vi "AVS_Read_Ch5-6-7.vi"(11 "refnum":refnum<file>) -> (1 "Resistance reading ch 5":dbl format="%.2f", 2 "Resistance reading ch 7":dbl format="%.2f", 3 "Resistance reading ch 6":dbl format="%.2f")   [LabVIEW 2016]
uses:
  Instrument_Setup_v2.vi
panel:
  in  "Delay (sec) 4":i16=1 min=0 max=3600 step=1
  in  "error in (no error) 5":errorcluster
  in  "error in (no error) 4":errorcluster
  in  "error in (no error) 3":errorcluster
  in  "Delay (sec) 3":i16=1 min=0 max=3600 step=1
  in  "Delay (sec) 2":i16=1 min=0 max=3600 step=1
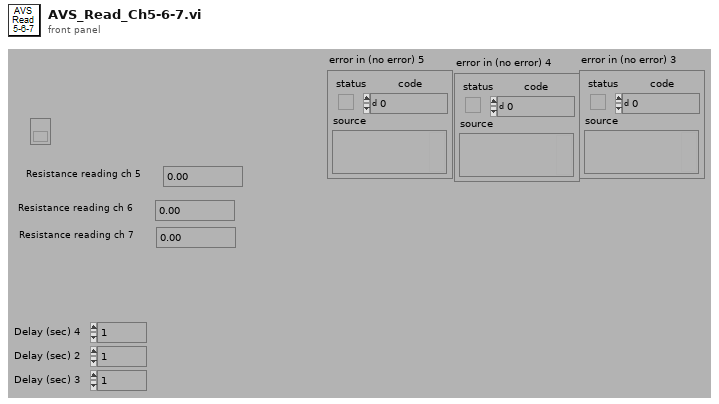
[diagram p1: front panel]
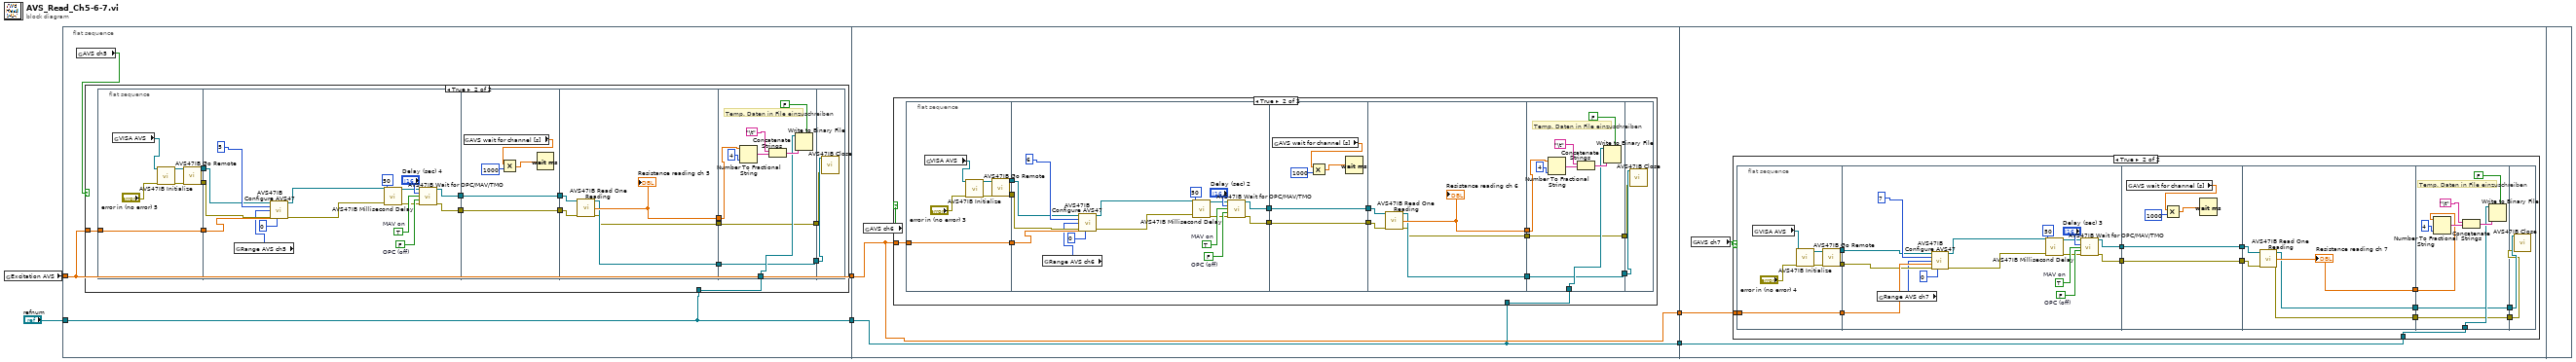
[diagram p0: block diagram]
diagram:
  n1 = global read "Instrument_Setup_v2.vi" "Excitation AVS"() -> (w5:dbl)
  n2 = flat-sequence {
    tunnel: "refnum" -> [w8]
    tunnel: w5 -> [w9]
    tunnel: [w9] -> w2
    tunnel: [w8] -> w1
    tunnel: [w69] -> w6
    tunnel: [w68] -> w3
    tunnel: w2 -> [w69]
    tunnel: w1 -> [w68]
    tunnel: w6 -> [w131]
    tunnel: w3 -> [w129]
    frame #0 {
      n3 = global read "Instrument_Setup_v2.vi" "AVS ch5"() -> (w7:bool)
      n4 = case shown="True" w7 {
        tunnel: w9 -> [_ w19]
        tunnel: w8 -> [_ w17]
        frame False {
        }
        frame True {
          n5 = flat-sequence {
            tunnel: w19 -> [w30]
            tunnel: [w30] -> w16
            tunnel: [w26] -> w15
            tunnel: [w25] -> w14
            tunnel: [w37] -> w23
            tunnel: [w36] -> w22
            tunnel: w16 -> [w34]
            tunnel: w15 -> [w33]
            tunnel: w14 -> [w32]
            tunnel: w23 -> [w51]
            tunnel: w22 -> [w50]
            tunnel: [w51] -> w21
            tunnel: [w50] -> w20
            tunnel: w21 -> [w56]
            tunnel: w20 -> [w55]
            tunnel: [w54] -> w18
            tunnel: [w53] -> w13
            tunnel: [w52] -> w10
            tunnel: w18 -> [w61]
            tunnel: w17 -> [w59]
            tunnel: w13 -> [w58]
            tunnel: [w58] -> w12
            tunnel: [w57] -> w11
            tunnel: w10 -> [w57]
            tunnel: w12 -> [w67]
            tunnel: w11 -> [w66]
            frame #0 {
              n6 = global read "Instrument_Setup_v2.vi" "VISA AVS"() -> (w24:refnum<visa-resource-name>)
              n7 = call "AVS47IB Initialize.vi"("VISA session"=w24, "error in (no error)"="error in (no error) 5") -> ("dup VISA session"=w28:refnum<visa-resource-name>, "error out"=w27:errorcluster)  [unwired: 12 in]
              n8 = call "AVS47IB Go Remote.vi"("VISA session"=w28, "error in (no error)"=w27) -> ("dup VISA session"=w26:refnum<visa-resource-name>, "error out"=w25:errorcluster)  [unwired: 12 in]
            }
            frame #1 {
              w44 = FALSE  # OPC (off)
              w45 = TRUE  # MAV on
              n9 = global read "Instrument_Setup_v2.vi" "Range AVS ch5"() -> (w31:i8)
              n10 = call "AVS47IB Configure AVS47.vi"("VISA session"=w33, "CHANNEL (-1:no change )"=i8 5, "RANGE  (-1:no change)"=w31, "EXCITATION (-1:no change)"=w34, "error in (no error)"=w32, "DISPLAY (-1:no change)"=i8 0) -> ("dup VISA session"=w39:refnum<visa-resource-name>, "error out"=w38:errorcluster)  [unwired: 8 in]
              n11 = call "AVS47IB Millisecond Delay.vi"("VISA session"=w39, "Delay (50 ms)"=50, "error in (no error)"=w38) -> ("dup VISA session"=w42:refnum<visa-resource-name>, "error out"=w41:errorcluster)  [unwired: 11 in]
              n12 = call "AVS47IB Wait for OPC/MAV/TMO.vi"("VISA session"=w42, "Timeout (2 sec)"="Delay (sec) 4", "MAV (on)"=w45, "OPC (off)"=w44, "error in (no error)"=w41) -> ("dup VISA session"=w37:refnum<visa-resource-name>, "error out"=w36:errorcluster)  [unwired: 8 in, 1 out]
            }
            frame #2 {
              n13 = global read "Instrument_Setup_v2.vi" "AVS wait for channel [s]"() -> (w49:dbl)
              n14 = Multiply(x=w49, y=1000) -> (x*y=w47:dbl)
              n15 = Wait (ms)(milliseconds to wait=w47) -> ()  [unwired: 1 out]
            }
            frame #3 {
              n16 = call "AVS47IB Read One Reading.vi"("VISA session"=w56, "error in (no error)"=w55) -> ("dup VISA session"=w53:refnum<visa-resource-name>, "Resistance reading"=w54:dbl, "error out"=w52:errorcluster)  [unwired: 9 in, 2 out]
              "Resistance reading ch 5" <- w54
            }
            frame #4 {
              # "Temp. Daten in File einzuschreiben"
              n17 = Number To Fractional String(number=w61, precision (6)=i16 4) -> (F-format string=w60:string)  [unwired: 2 in]
              n18 = Concatenate Strings("\t", w60) -> (w65:string)
              n19 = Write to Binary File ("Write File")(file (use dialog)=w59, data=w65, 5:FALSE ("prepend array or string size? (T)")) -> ()  [unwired: 3 in, 3 out]
            }
            frame #5 {
              n20 = call "AVS47IB Close.vi"("VISA session"=w67, "error in (no error)"=w66) -> ()  [unwired: 13 in, 1 out]
            }
          }
        }
      }
    }
    frame #1 {
      n21 = global read "Instrument_Setup_v2.vi" "AVS ch6"() -> (w70:bool)
      n22 = case shown="True" w70 {
        tunnel: w69 -> [_ w80]
        tunnel: w68 -> [_ w78]
        frame False {
        }
        frame True {
          n23 = flat-sequence {
            tunnel: w80 -> [w91]
            tunnel: [w91] -> w77
            tunnel: [w87] -> w76
            tunnel: [w86] -> w75
            tunnel: [w98] -> w84
            tunnel: [w97] -> w83
            tunnel: w77 -> [w95]
            tunnel: w76 -> [w94]
            tunnel: w75 -> [w93]
            tunnel: w84 -> [w112]
            tunnel: w83 -> [w111]
            tunnel: [w112] -> w82
            tunnel: [w111] -> w81
            tunnel: w82 -> [w117]
            tunnel: w81 -> [w116]
            tunnel: [w115] -> w79
            tunnel: [w114] -> w74
            tunnel: [w113] -> w71
            tunnel: w79 -> [w122]
            tunnel: w78 -> [w120]
            tunnel: w74 -> [w119]
            tunnel: [w119] -> w73
            tunnel: [w118] -> w72
            tunnel: w71 -> [w118]
            tunnel: w73 -> [w128]
            tunnel: w72 -> [w127]
            frame #0 {
              n24 = global read "Instrument_Setup_v2.vi" "VISA AVS"() -> (w85:refnum<visa-resource-name>)
              n25 = call "AVS47IB Initialize.vi"("VISA session"=w85, "error in (no error)"="error in (no error) 3") -> ("dup VISA session"=w89:refnum<visa-resource-name>, "error out"=w88:errorcluster)  [unwired: 12 in]
              n26 = call "AVS47IB Go Remote.vi"("VISA session"=w89, "error in (no error)"=w88) -> ("dup VISA session"=w87:refnum<visa-resource-name>, "error out"=w86:errorcluster)  [unwired: 12 in]
            }
            frame #1 {
              w105 = FALSE  # OPC (off)
              w106 = TRUE  # MAV on
              n27 = global read "Instrument_Setup_v2.vi" "Range AVS ch6"() -> (w92:i8)
              n28 = call "AVS47IB Configure AVS47.vi"("VISA session"=w94, "CHANNEL (-1:no change )"=i8 6, "RANGE  (-1:no change)"=w92, "EXCITATION (-1:no change)"=w95, "error in (no error)"=w93, "DISPLAY (-1:no change)"=i8 0) -> ("dup VISA session"=w100:refnum<visa-resource-name>, "error out"=w99:errorcluster)  [unwired: 8 in]
              n29 = call "AVS47IB Millisecond Delay.vi"("VISA session"=w100, "Delay (50 ms)"=50, "error in (no error)"=w99) -> ("dup VISA session"=w103:refnum<visa-resource-name>, "error out"=w102:errorcluster)  [unwired: 11 in]
              n30 = call "AVS47IB Wait for OPC/MAV/TMO.vi"("VISA session"=w103, "Timeout (2 sec)"="Delay (sec) 2", "MAV (on)"=w106, "OPC (off)"=w105, "error in (no error)"=w102) -> ("dup VISA session"=w98:refnum<visa-resource-name>, "error out"=w97:errorcluster)  [unwired: 8 in, 1 out]
            }
            frame #2 {
              n31 = global read "Instrument_Setup_v2.vi" "AVS wait for channel [s]"() -> (w110:dbl)
              n32 = Multiply(x=w110, y=1000) -> (x*y=w108:dbl)
              n33 = Wait (ms)(milliseconds to wait=w108) -> ()  [unwired: 1 out]
            }
            frame #3 {
              n34 = call "AVS47IB Read One Reading.vi"("VISA session"=w117, "error in (no error)"=w116) -> ("dup VISA session"=w114:refnum<visa-resource-name>, "Resistance reading"=w115:dbl, "error out"=w113:errorcluster)  [unwired: 9 in, 2 out]
              "Resistance reading ch 6" <- w115
            }
            frame #4 {
              # "Temp. Daten in File einzuschreiben"
              n35 = Number To Fractional String(number=w122, precision (6)=i16 4) -> (F-format string=w121:string)  [unwired: 2 in]
              n36 = Concatenate Strings("\t", w121) -> (w126:string)
              n37 = Write to Binary File ("Write File")(file (use dialog)=w120, data=w126, 5:FALSE ("prepend array or string size? (T)")) -> ()  [unwired: 3 in, 3 out]
            }
            frame #5 {
              n38 = call "AVS47IB Close.vi"("VISA session"=w128, "error in (no error)"=w127) -> ()  [unwired: 13 in, 1 out]
            }
          }
        }
      }
    }
    frame #2 {
      n39 = global read "Instrument_Setup_v2.vi" "AVS ch7"() -> (w130:bool)
      n40 = case shown="True" w130 {
        tunnel: w131 -> [_ w141]
        tunnel: w129 -> [_ w139]
        frame False {
        }
        frame True {
          n41 = flat-sequence {
            tunnel: w141 -> [w152]
            tunnel: [w152] -> w138
            tunnel: [w148] -> w137
            tunnel: [w147] -> w136
            tunnel: [w159] -> w145
            tunnel: [w158] -> w144
            tunnel: w138 -> [w156]
            tunnel: w137 -> [w154]
            tunnel: w136 -> [w155]
            tunnel: w145 -> [w173]
            tunnel: w144 -> [w172]
            tunnel: [w173] -> w143
            tunnel: [w172] -> w142
            tunnel: w143 -> [w178]
            tunnel: w142 -> [w177]
            tunnel: [w176] -> w140
            tunnel: [w175] -> w135
            tunnel: [w174] -> w132
            tunnel: w140 -> [w182]
            tunnel: w139 -> [w181]
            tunnel: w135 -> [w180]
            tunnel: [w180] -> w134
            tunnel: [w179] -> w133
            tunnel: w132 -> [w179]
            tunnel: w134 -> [w189]
            tunnel: w133 -> [w188]
            frame #0 {
              n42 = global read "Instrument_Setup_v2.vi" "VISA AVS"() -> (w146:refnum<visa-resource-name>)
              n43 = call "AVS47IB Initialize.vi"("VISA session"=w146, "error in (no error)"="error in (no error) 4") -> ("dup VISA session"=w150:refnum<visa-resource-name>, "error out"=w149:errorcluster)  [unwired: 12 in]
              n44 = call "AVS47IB Go Remote.vi"("VISA session"=w150, "error in (no error)"=w149) -> ("dup VISA session"=w148:refnum<visa-resource-name>, "error out"=w147:errorcluster)  [unwired: 12 in]
            }
            frame #1 {
              w166 = FALSE  # OPC (off)
              w167 = TRUE  # MAV on
              n45 = global read "Instrument_Setup_v2.vi" "Range AVS ch7"() -> (w153:i8)
              n46 = call "AVS47IB Configure AVS47.vi"("VISA session"=w154, "CHANNEL (-1:no change )"=i8 7, "RANGE  (-1:no change)"=w153, "EXCITATION (-1:no change)"=w156, "error in (no error)"=w155, "DISPLAY (-1:no change)"=i8 0) -> ("dup VISA session"=w161:refnum<visa-resource-name>, "error out"=w160:errorcluster)  [unwired: 8 in]
              n47 = call "AVS47IB Millisecond Delay.vi"("VISA session"=w161, "Delay (50 ms)"=50, "error in (no error)"=w160) -> ("dup VISA session"=w164:refnum<visa-resource-name>, "error out"=w163:errorcluster)  [unwired: 11 in]
              n48 = call "AVS47IB Wait for OPC/MAV/TMO.vi"("VISA session"=w164, "Timeout (2 sec)"="Delay (sec) 3", "MAV (on)"=w167, "OPC (off)"=w166, "error in (no error)"=w163) -> ("dup VISA session"=w159:refnum<visa-resource-name>, "error out"=w158:errorcluster)  [unwired: 8 in, 1 out]
            }
            frame #2 {
              n49 = global read "Instrument_Setup_v2.vi" "AVS wait for channel [s]"() -> (w171:dbl)
              n50 = Multiply(x=w171, y=1000) -> (x*y=w169:dbl)
              n51 = Wait (ms)(milliseconds to wait=w169) -> ()  [unwired: 1 out]
            }
            frame #3 {
              n52 = call "AVS47IB Read One Reading.vi"("VISA session"=w178, "error in (no error)"=w177) -> ("dup VISA session"=w175:refnum<visa-resource-name>, "Resistance reading"=w176:dbl, "error out"=w174:errorcluster)  [unwired: 9 in, 2 out]
              "Resistance reading ch 7" <- w176
            }
            frame #4 {
              # "Temp. Daten in File einzuschreiben"
              n53 = Number To Fractional String(number=w182, precision (6)=i16 4) -> (F-format string=w183:string)  [unwired: 2 in]
              n54 = Concatenate Strings("\t", w183) -> (w187:string)
              n55 = Write to Binary File ("Write File")(file (use dialog)=w181, data=w187, 5:FALSE ("prepend array or string size? (T)")) -> ()  [unwired: 3 in, 3 out]
            }
            frame #5 {
              n56 = call "AVS47IB Close.vi"("VISA session"=w189, "error in (no error)"=w188) -> ()  [unwired: 13 in, 1 out]
            }
          }
        }
      }
    }
    frame #3 {
    }
  }
